vi "PID control - Copy.vi"() -> ()   [LabVIEW 2017]
uses:
  <vilib>/Simulation/Scripting/Companion Diagram/SimConfigNode/SimParams.ctl
  <vilib>/Simulation/Scripting/Companion Diagram/SimConfigNode/_simSolvers.ctl
  <vilib>/Simulation/Implementation/Shared/SIMSCR Execution Mode.ctl
  <vilib>/Simulation/Param Hierarchy/Typedefs/SIMPH Param Control Actions.ctl
  <vilib>/Simulation/Implementation/Shared/NILVSim_ParamChanged.vi
  <vilib>/Simulation/Implementation/Shared/NILVSIM_BeginStep.vi
  <vilib>/Simulation/Implementation/Shared/NILVSim_Manager.vi
  <vilib>/Utility/error.llb/Clear Errors.vi
  <vilib>/Simulation/Implementation/Shared/NILVSim_FinalizeModel.vi
  <vilib>/DAQmx/read.llb/DAQmx Read (Counter DBL 1Chan 1Samp).vi
  <vilib>/DAQmx/read.llb/DAQmx Read (Digital Bool 1Line 1Point).vi
  917b7e52-755f-4d44-bea8-9e7c9beac24e.vi
  a58f9967-76f1-4ebc-ad3d-26e75a3ca160.vi
  <vilib>/DAQmx/write.llb/DAQmx Write (Analog DBL 1Chan 1Samp).vi
  <vilib>/DAQmx/create/channels.llb/DAQmx Create Channel (AO-Voltage-Basic).vi
  <vilib>/DAQmx/create/channels.llb/DAQmx Create Channel (DI-Digital Input).vi
  <vilib>/DAQmx/create/channels.llb/DAQmx Create Channel (CI-Count Edges).vi
  <vilib>/Simulation/Implementation/Shared/SIM Unbundle Sim Info.vi
  <vilib>/Simulation/Implementation/Shared/NILVSim_Initialize.vi
  <vilib>/Simulation/Utility/Implementation/NILVSim Get Time and IsAcceptedStep.vi
  <vilib>/Simulation/Implementation/Shared/SIMSH Read Queue.vi
  <vilib>/Simulation/Implementation/Shared/NILVSim_GetModelError.vi
  <vilib>/Simulation/Implementation/Shared/SIM Bundle Sim Info.vi
  <vilib>/DAQmx/miscellaneous.llb/DAQmx Fill In Error Info.vi
  <vilib>/Simulation/Implementation/XNodeFramework/SimXNode/SimX.xnode
  <vilib>/Simulation/Model Libraries/PID/SIM PID (Parallel).vi
  <vilib>/Simulation/Model Libraries/PID/SIM PID.vi
  <vilib>/Simulation/Scripting/Companion Diagram/SimConfigNode/SimDog.xnode
  <vilib>/Simulation/Model Libraries/PID/SIM PID (Academic).vi
  <vilib>/Simulation/Implementation/Shared/NI_SIM_Implementation.lvlib
panel:
  out "resetting x":bool
  out "resetting y":bool
  out "index":dbl
  out "x check":dbl
  out "stop":bool
  out "y final check":dbl
  out "y check":dbl
  out "array x Length":dbl
  out "X array":dbl[](array[numeric])
  out "array Y length":dbl
  out "Y array":dbl[](array[numeric])
  out "Numeric y":dbl
  out "Numeric x":dbl
  out "Numeric 2":dbl
  in  "Radius":dbl
  out "led check":bool
  in  "check instruc":bool
  out "down 2":bool
  out "down":bool
  out "right":bool
  out "x entered":dbl
  out "y enetred":dbl
  out "greater -1 x":bool
  out "less 1 x":bool
  out "direction selected":dbl
  out "circle reset":bool
  in  "part circle":T1(ring)=enum."a"
  out "at 2f":bool
  out "Step 2J":bool
  out "Step 2H":bool
  out "Shape drawing steps":enum16{"corner", "1st switch", "reverse"}(ring)
  out "Step 2D":bool
  out "Step 2C":bool
  out "c":bool
  in  "height":dbl
  in  "length":dbl
  in  "part":T2(ring)=enum."a"
  out "Step 2A":bool
  out "Step 2B":bool
  in  "Has encoders been reset?":enum16{"don't reset", "reset"}(ring)
  out "x distance currently being travelled":dbl
  out "y distance currently being travelled":dbl
  out "error calced":dbl
  out "p1 dis 2":dbl
  out "p1 dis":dbl
  out "error y":dbl
  out "calc distance y":dbl
  out "calc distanc x":dbl
  out "error x":dbl
  out "reached y":bool
  out "reached x":bool
  out "Numeric":dbl
  in  "Draw rectangle":bool
  in  "Draw circle":bool
  out "In drawing mode":bool
  in  "Right-Down":bool
  in  "Left-Up":bool
  in  "Left-Down":bool
  in  "Right-Up":bool
  in  "right":bool
  in  "left":bool
  in  "motor 2":dbl(slide)=1.5 scale=-10.0..10.0
  in  "down":bool
  in  "up":bool
  in  "Y Length":dbl=30.0
  in  "X Length":dbl=30.0
  in  "Motor 2 encoder":tag="Dev1/ctr1"
  out "Pulses M2":dbl format="%.2f"
  in  "Motor 1 encoder":tag="Dev1/ctr0"
  out "Pulses M1":dbl format="%.2f"
  out "Right":bool
  out "Bottom":bool
  out "Left":bool
  out "Top":bool
  in  "Switch 4/Line 3":tag="Dev1/port0/line3"
  in  "Switch 3/Line 2":tag="Dev1/port0/line2"
  in  "Switch 2/Line 1":tag="Dev1/port0/line1"
  in  "Switch 1/Line 0":tag="Dev1/port0/line0"
  in  "Motor stop":bool
  in  "Motor 1":tag="Dev1/ao0"
  in  "max Voltage":dbl=10.0
  in  "Min Voltage":dbl=-10.0
  in  "Motor 2":tag="Dev1/ao1"
  in  "motor 1":dbl(slide)=1.5 scale=-10.0..10.0
  in  "stop":bool
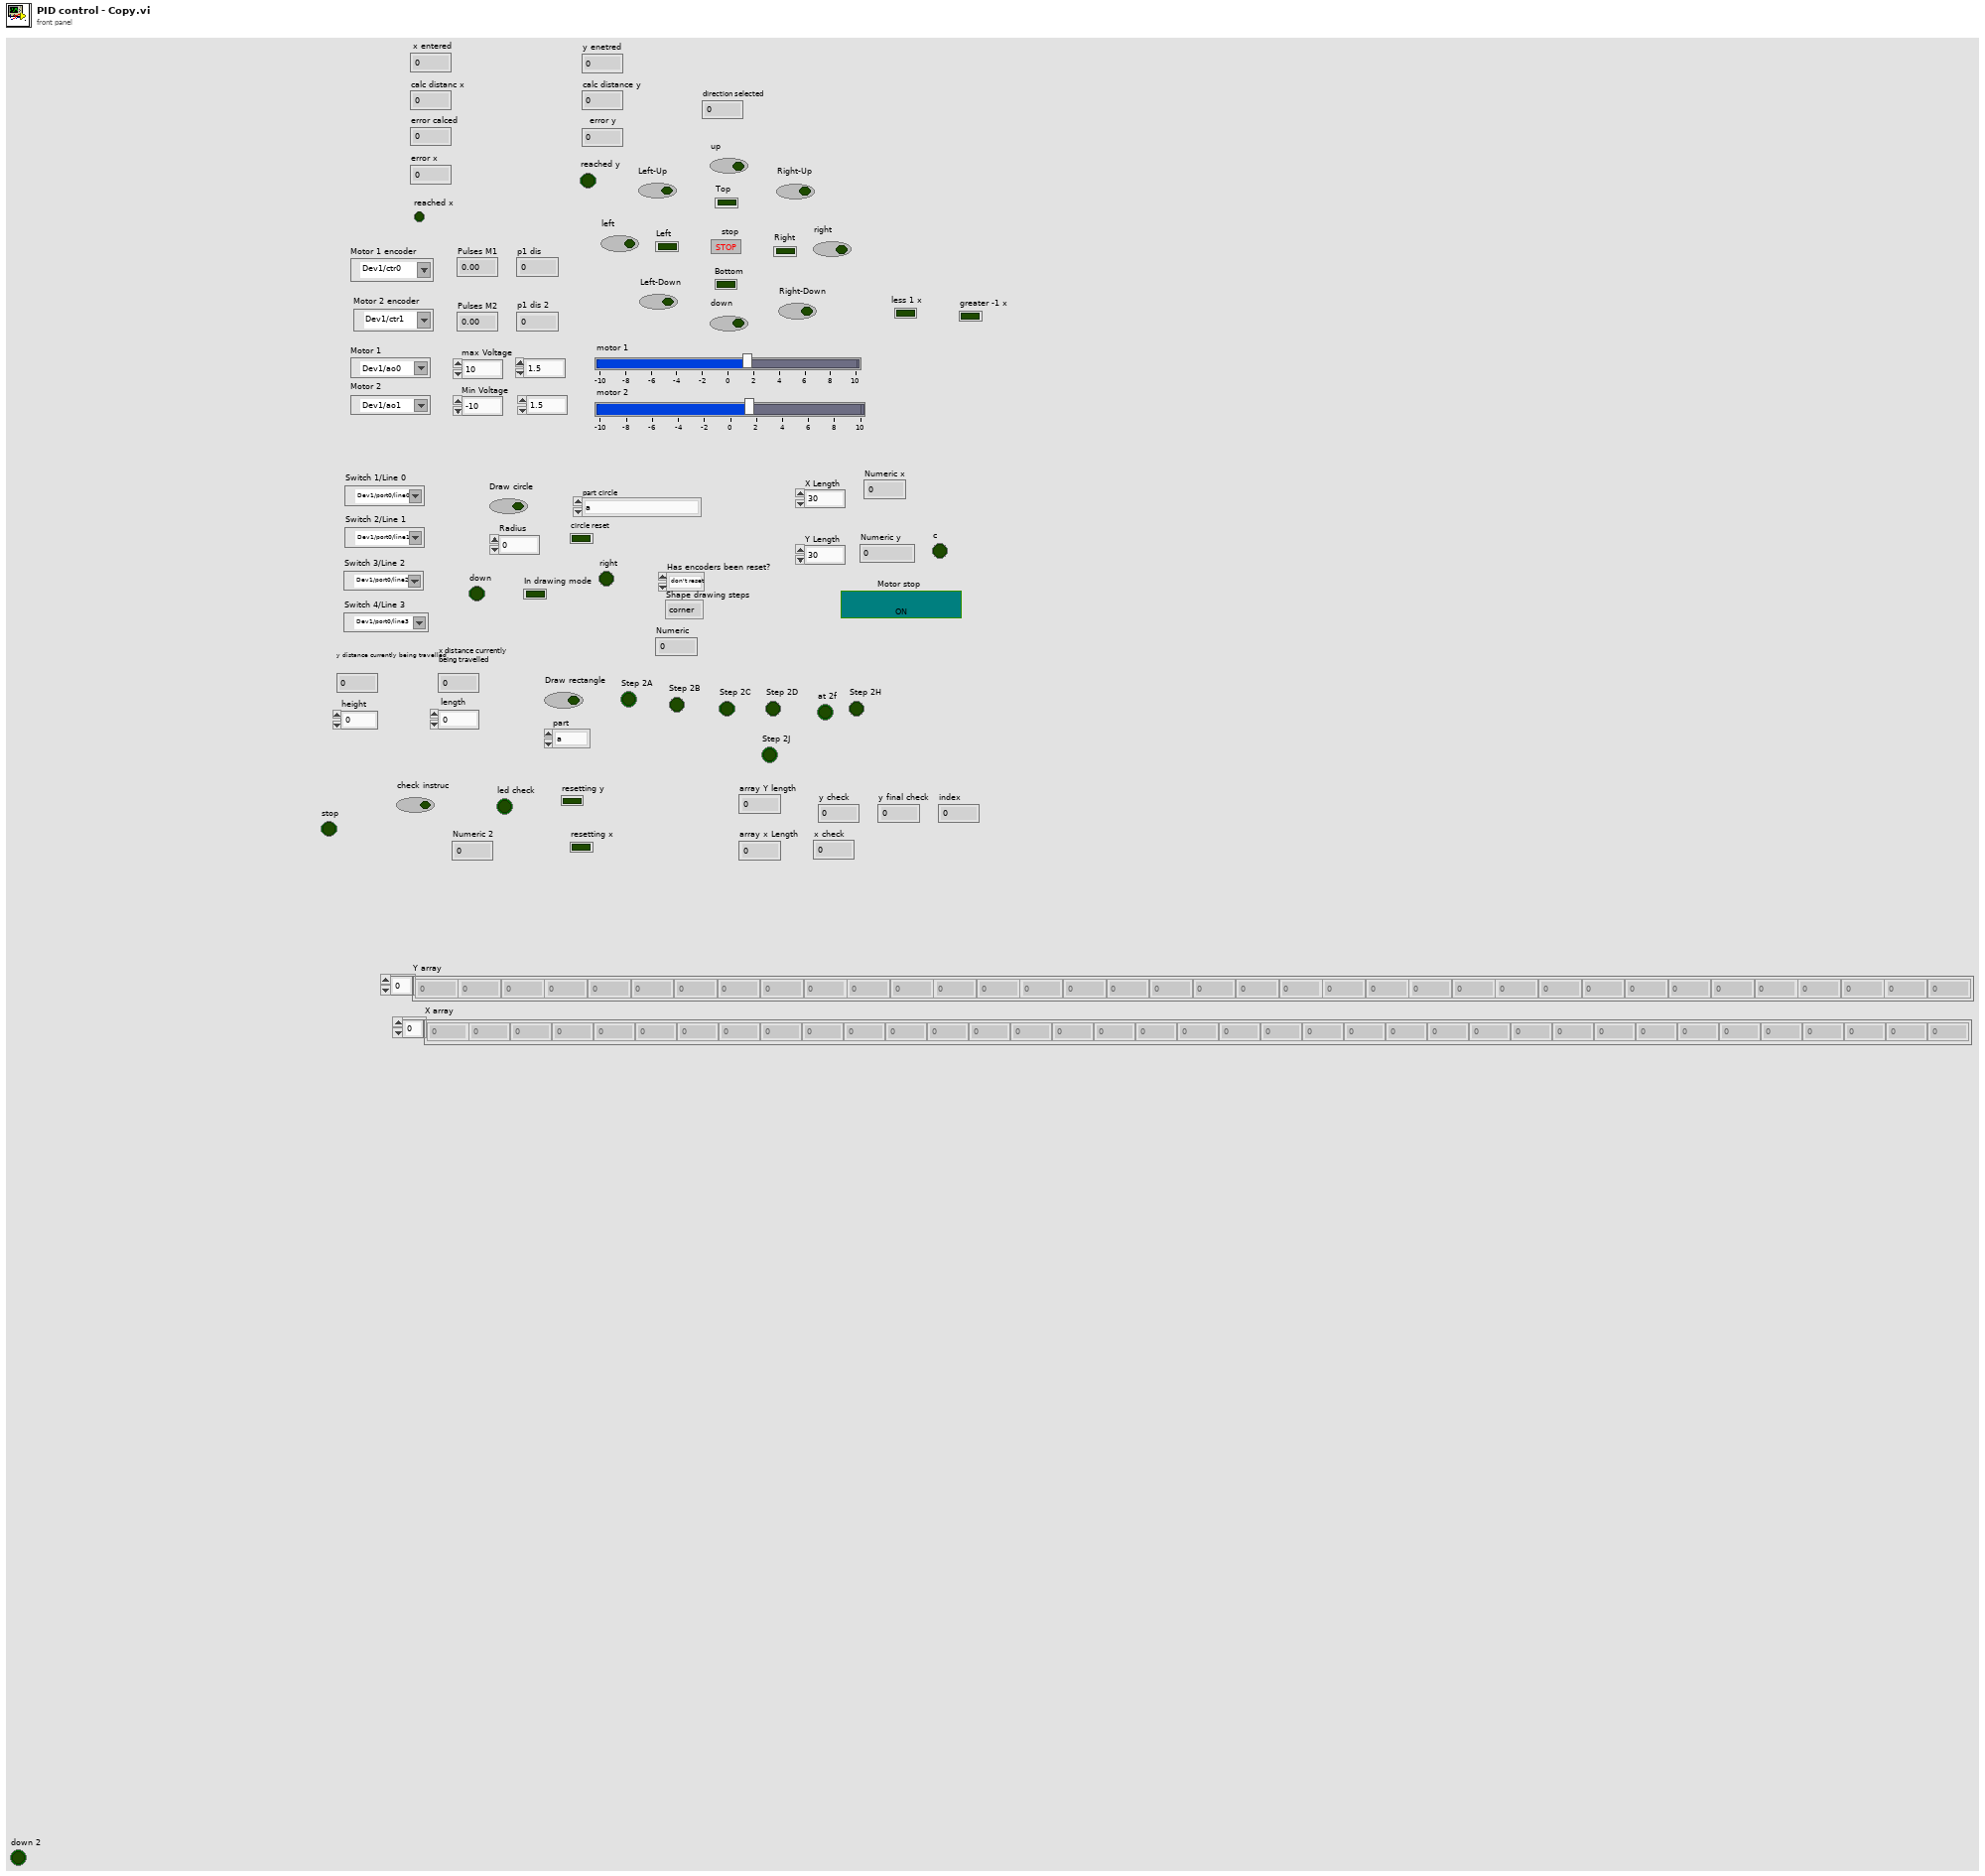
[diagram p1: front panel]
types:
  T1 = enum16{"nothing", "circle", "reset_before_circle", "radius_travel", "going right", "going down", "a"}
  T2 = enum16{"nothing", "j", "i", "h", "g", "f", "e", "d", "c", "b", "a"}
  T3 = enum16{"Simulate to Completion", "Single Time-Step Simulation (Fixed Step Only)"}
  T4 = typedef "SIMSCR Execution Mode.ctl" = enum16{"Simulate to Completion", "Single Time-Step Simulation (Fixed Step Only)"}
  T5 = typedef "SIMPH Param Control Actions.ctl" = enum16{"get params", "set params"}
  T6 = cluster{"SIMSH Sim Time":dbl, "SIM PID Derivative Gain.vi":cluster{"output":dbl}, "SIM PID Derivative Gain.vi - SIMSH":cluster{"SIMSH Sim Time":dbl, "t 3":dbl, "Select 2":cluster{"s? t:f":dbl}, "Equal?":cluster{"x = y?":bool}, "Or":cluster{"x .or. y?":bool}, "Equal To 0?":cluster{"x = 0?":bool}}, "High Frequency [s] (Tf)":dbl, "Gain":cluster{"output":dbl}, "Summation":cluster{"Result":dbl}, "Integral Gain - series.vi":cluster{"output":dbl}, "Integral Gain - series.vi - SIMSH":cluster{"SIMSH Sim Time":dbl, "Select 2":cluster{"s? t:f":dbl}, "integral in gain?":bool, "Integrator":cluster{"output y(t)":dbl}, "Gain 2":cluster{"output":dbl}, "Select":cluster{"s? t:f":dbl}, "Equal To 0?":cluster{"x = 0?":bool}, "Reciprocal":cluster{"1/x":dbl}}}
  T7 = typedef "SimParams.ctl" = cluster{"Initial Time (s)":dbl, "Final Time (s)":dbl, "Step Size (s)":dbl, "ODE Solver":T8, "Minimum Step Size (s)":dbl, "Maximum Step Size (s)":dbl, "Relative Tolerance":dbl, "Absolute Tolerance":dbl, "Software Timing":bool, "Initial Step Size (s)":dbl, "Automatic Fixed Step Size?":bool, "Automatic Discrete Step Size?":bool, "Discrete Step Size (s)":dbl, "Calculate using Time Step":bool, "Solver Wired?":bool, "Prev.Frm.Expected End":u64, "Prev.Frm.Actual End":u64, "Prev.Frm.Finished Late?":bool, "Prev.Iter.Expected End":u64, "Prev.Iter.Actual End":u64, "Prev.Iter.Finished Late?":bool, "Expected Iteration Start":u64, "Actual Iteration Start":u64, "Expected Frame Start":u64, "Actual Frame Start":u64, "Source Name":string, "Name":string, "Period":i64, "Deadline":i64, "Offset":i64, "Start":i64, "Priority":i32, "Timeout":i32, "Processor":i32, "Mode":enum32{"No Change", "Process missed periods, maintain original phase", "Discard missed periods, maintain original phase", "Process missed periods, ignore original phase", "Discard missed periods, ignore original phase"}, "Wakeup reason":enum32{"Normal", "Aborted", "Asynchronous wakeup", "Timing source error", "Timed loop error", "Timeout"}, "Error":errorcluster, "Source Type":string, "Secondary Source Type":string, "Global End Time":u64, "Global Start Time":u64, "Full Solver Reset":bool, "Execution Mode":T4, "Nan/Inf Check":bool, "Custom Solver Library":string, "Solver Is Variable":bool, "custom solver name":string, "Signal Collection Decimation":u32}
  T8 = typedef "_simSolvers.ctl" = enum16{"Runge-Kutta 1 (Euler)", "Runge-Kutta 2", "Runge-Kutta 3", "Runge-Kutta 4", "Runge-Kutta 23 (variable)", "Runge-Kutta 45 (variable)", "BDF (variable)", "Adams-Moulton (variable)", "Rosenbrock (variable)", "Discrete States Only", "SDIRK 4 (variable)", "Radau 5 (variable)", "Radau 9 (variable)", "Radau 13 (variable)", "Radau [Variable Order] (variable)", "Gear's Method (variable)", "Linearizer", "State Query", "Trim Eval", "Custom Solver"}
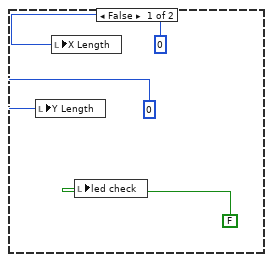
[diagram p2: hidden frame]
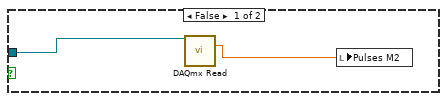
[diagram p3: hidden frame]
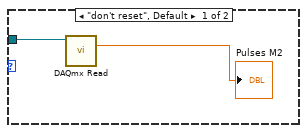
[diagram p4: hidden frame]
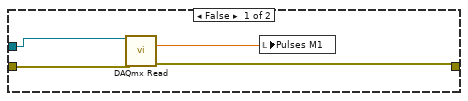
[diagram p5: hidden frame]
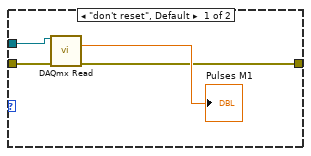
[diagram p6: hidden frame]
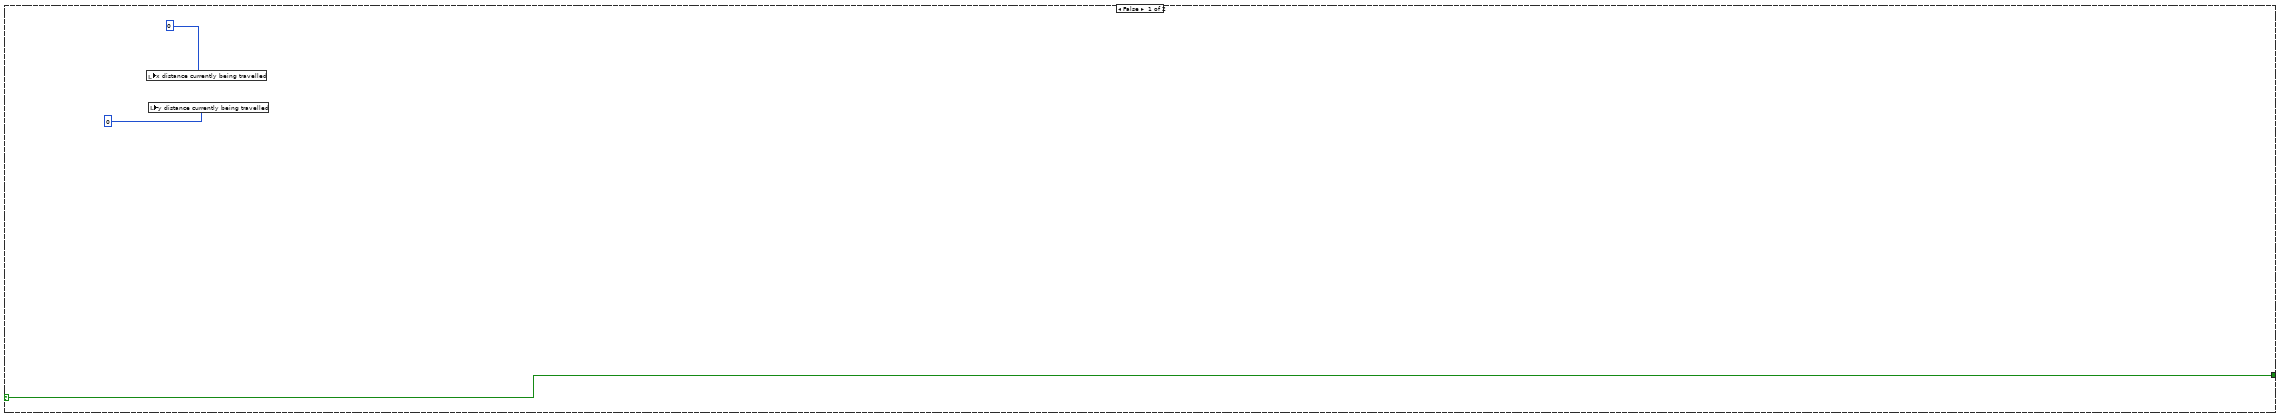
[diagram p7: hidden frame]
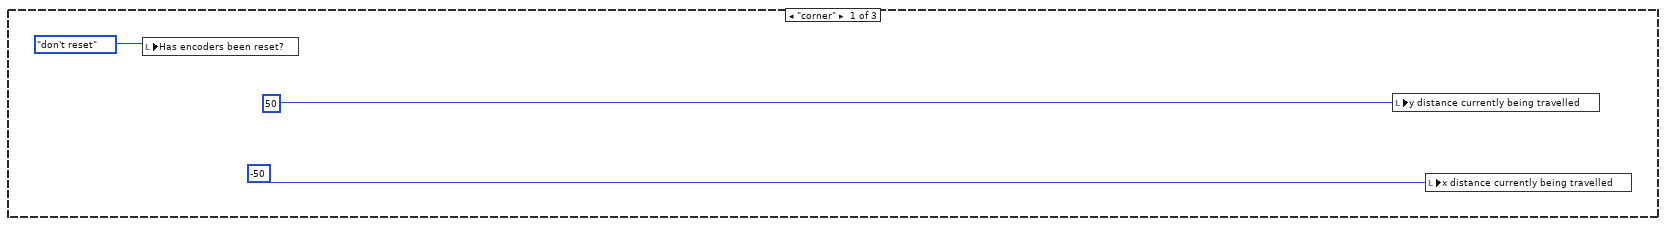
[diagram p8: hidden frame]
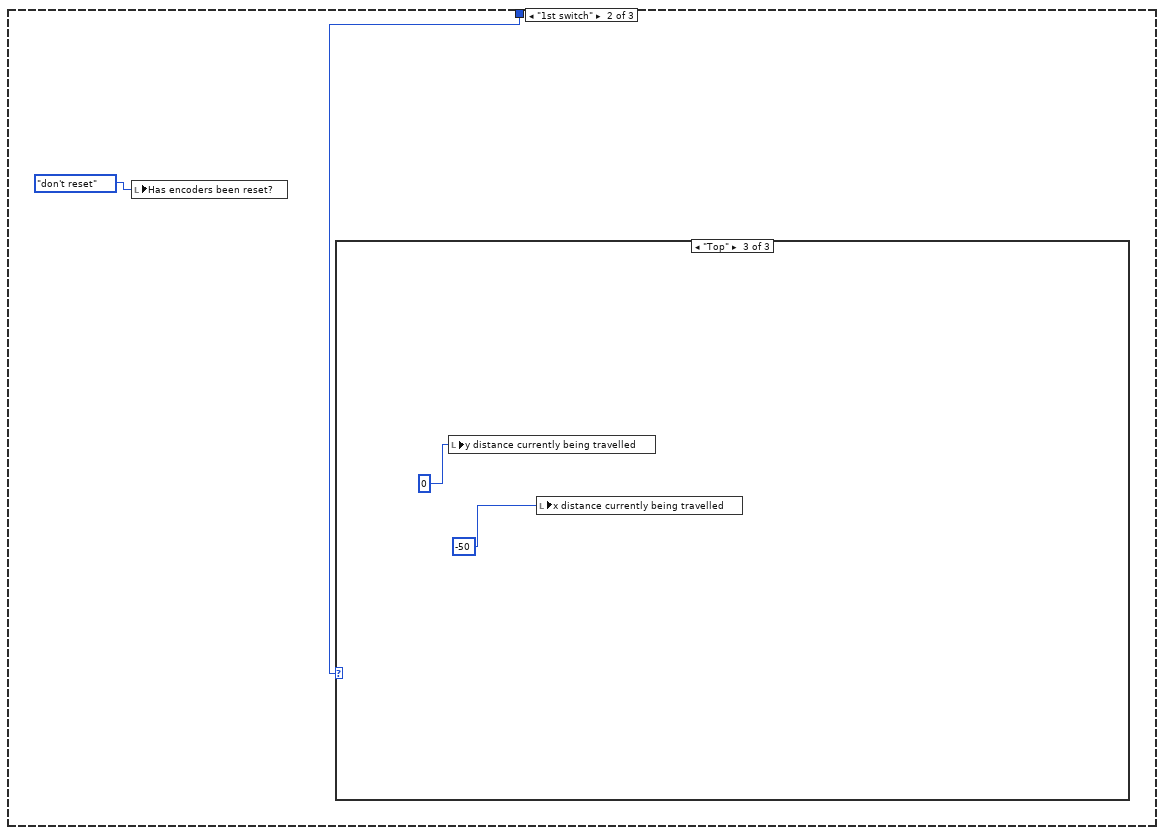
[diagram p9: hidden frame]
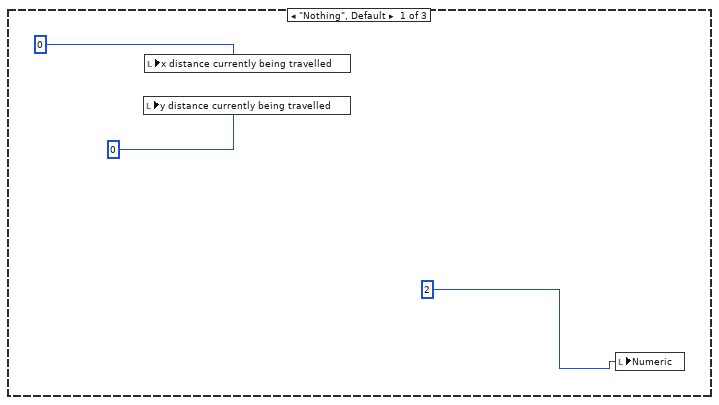
[diagram p10: hidden frame]
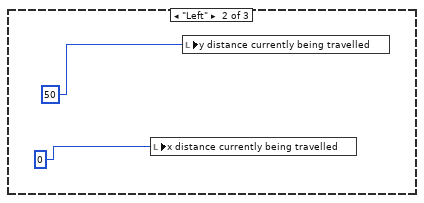
[diagram p11: hidden frame]
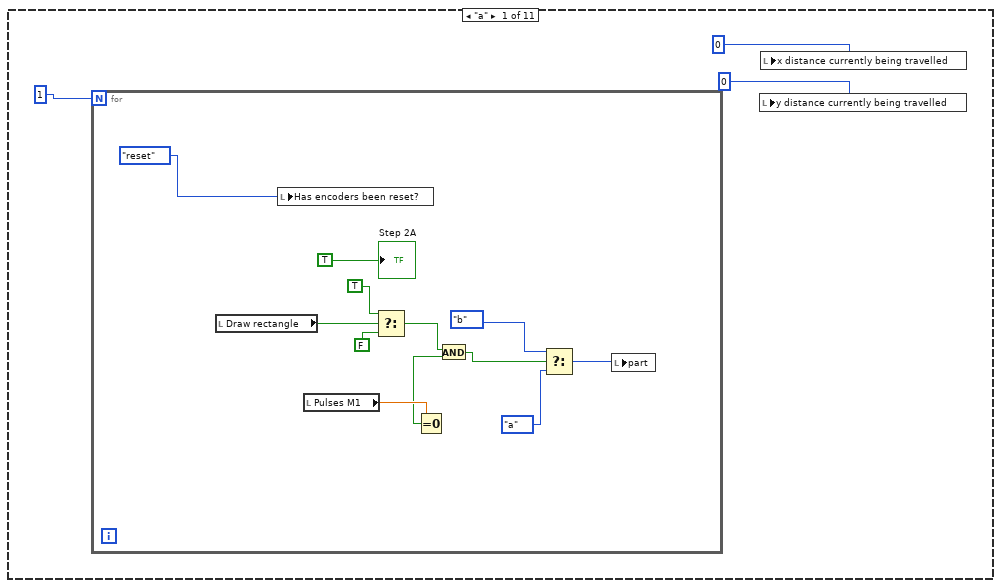
[diagram p12: hidden frame]
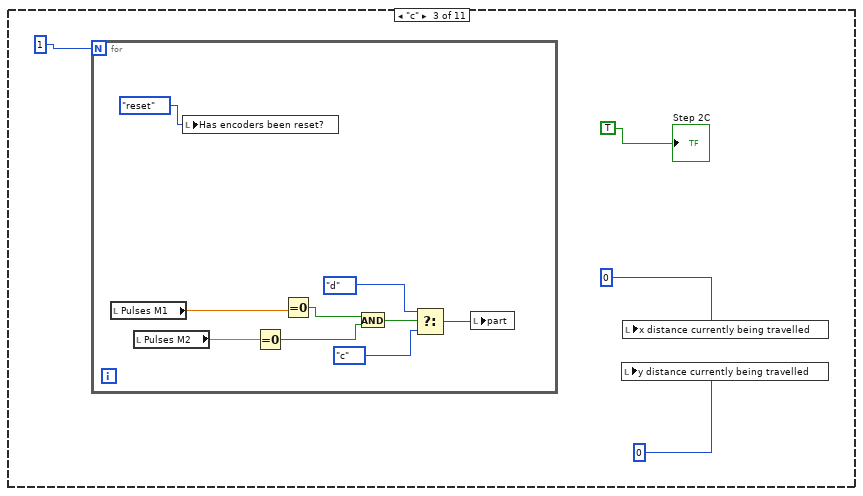
[diagram p13: hidden frame]
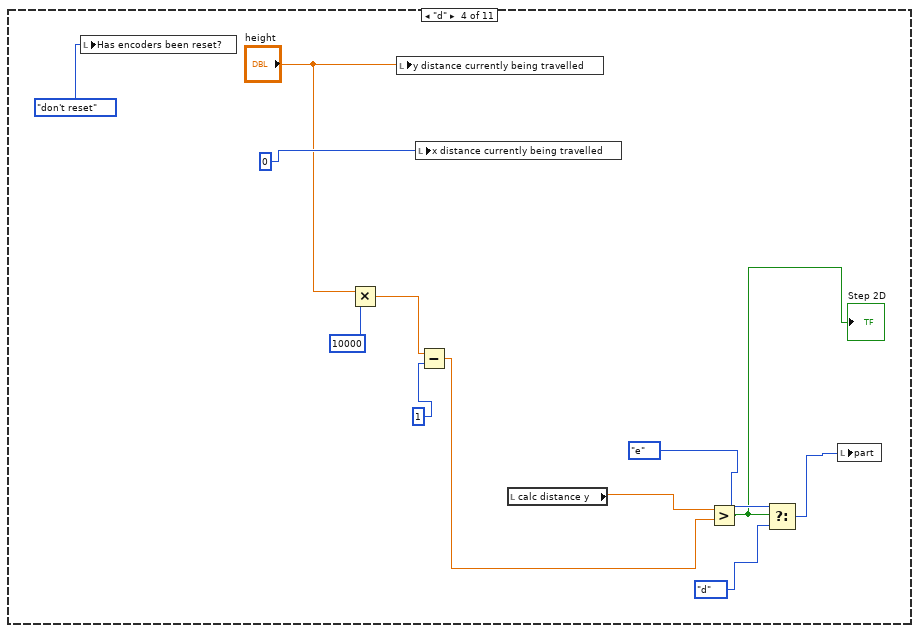
[diagram p14: hidden frame]
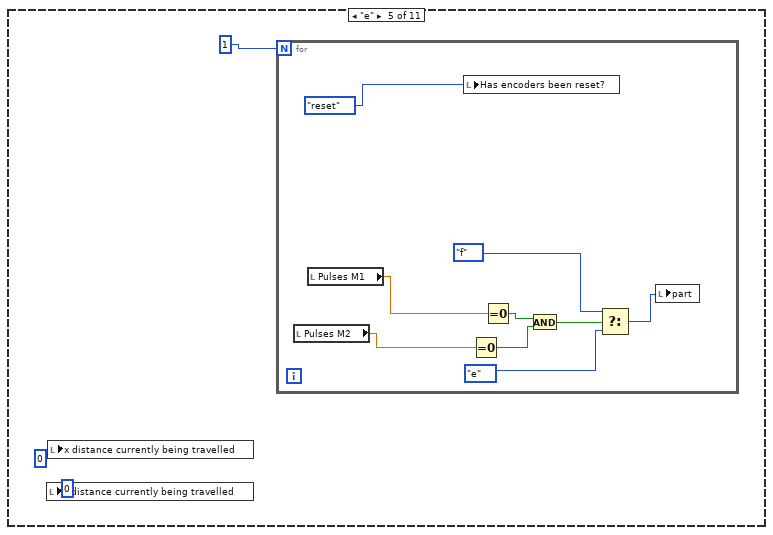
[diagram p15: hidden frame]
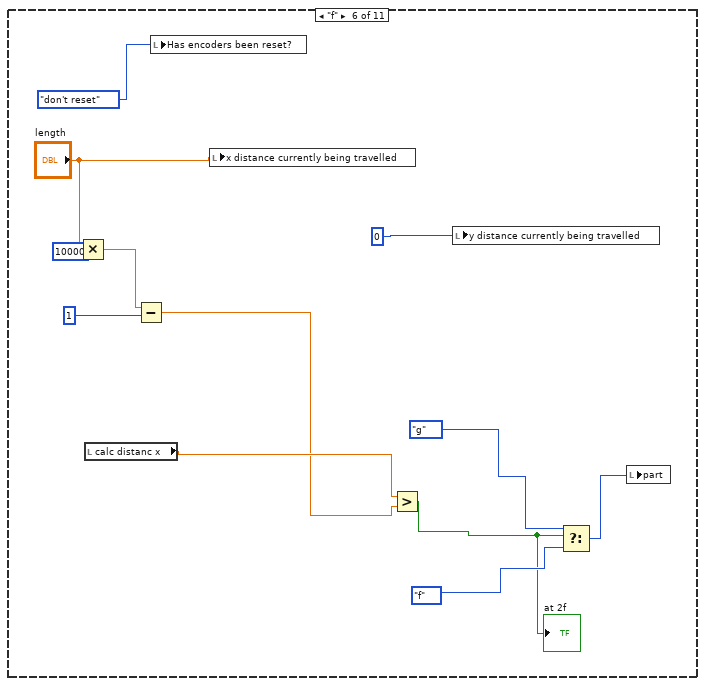
[diagram p16: hidden frame]
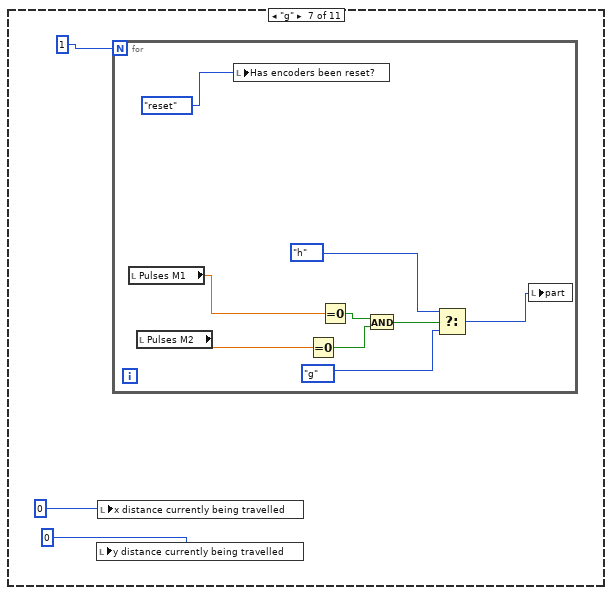
[diagram p17: hidden frame]
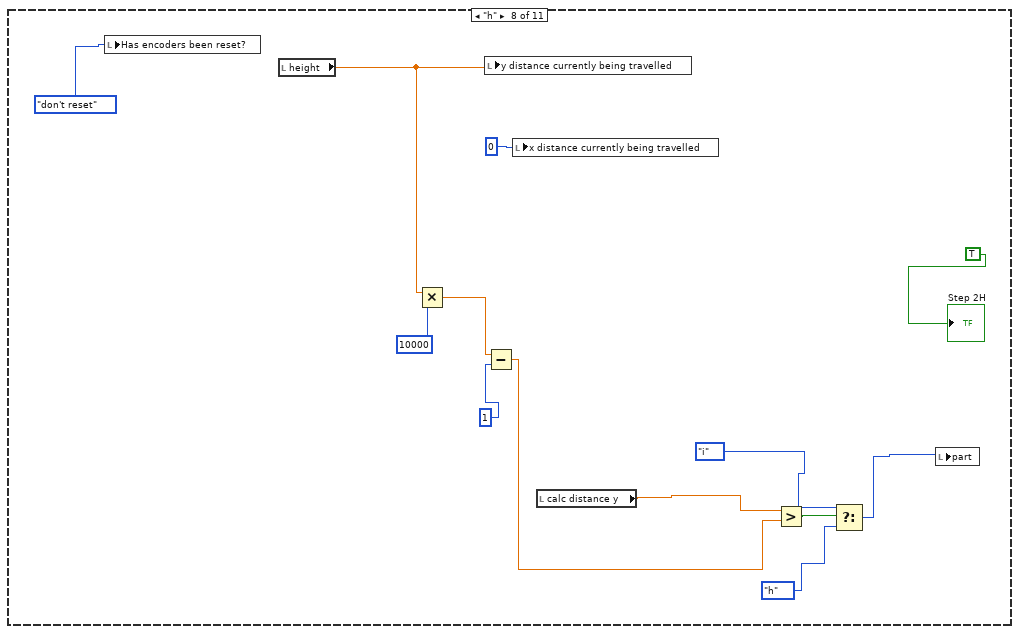
[diagram p18: hidden frame]
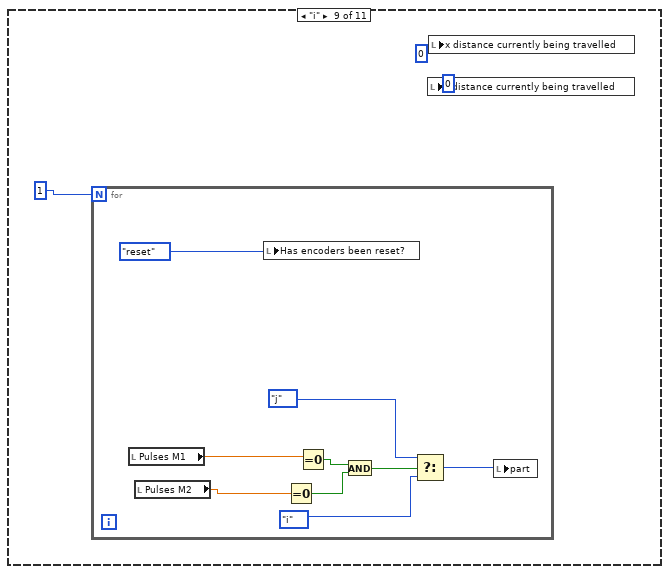
[diagram p19: hidden frame]
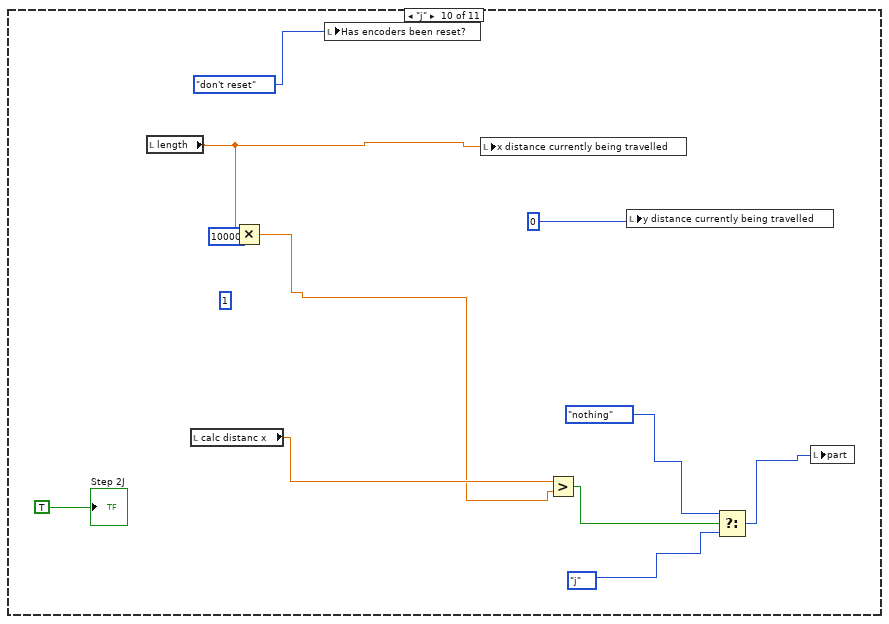
[diagram p20: hidden frame]
diagram:
  n1 = call-poly <vilib>:"DAQmx Create Virtual Channel.vi"("lines"="Switch 1/Line 0") -> ("task out"=w36:refnum<k21>, "error out"=w32:errorcluster)  [unwired: 13 in]
  n2 = call-poly <vilib>:"DAQmx Create Virtual Channel.vi"("lines"="Switch 2/Line 1") -> ("task out"=w35:refnum<k21>, "error out"=w31:errorcluster)  [unwired: 13 in]
  n3 = call-poly <vilib>:"DAQmx Create Virtual Channel.vi"("lines"="Switch 3/Line 2") -> ("task out"=w34:refnum<k21>, "error out"=w30:errorcluster)  [unwired: 13 in]
  n4 = call-poly <vilib>:"DAQmx Create Virtual Channel.vi"("lines"="Switch 4/Line 3") -> ("task out"=w33:refnum<k21>, "error out"=w29:errorcluster)  [unwired: 13 in]
  n5 = call <vilib>:"DAQmx Start Task.vi"("task/channels in"=w36, "error in"=w32) -> ("task out"=w28:refnum<k21>, "error out"=w26:errorcluster)  [unwired: 12 in]
  n6 = call <vilib>:"DAQmx Start Task.vi"("task/channels in"=w35, "error in"=w31) -> ("task out"=w24:refnum<k21>, "error out"=w21:errorcluster)  [unwired: 12 in]
  n7 = call <vilib>:"DAQmx Start Task.vi"("task/channels in"=w34, "error in"=w30) -> ("task out"=w23:refnum<k21>, "error out"=w20:errorcluster)  [unwired: 12 in]
  n8 = call <vilib>:"DAQmx Start Task.vi"("task/channels in"=w33, "error in"=w29) -> ("task out"=w22:refnum<k21>, "error out"=w19:errorcluster)  [unwired: 12 in]
  n9 = call-poly <vilib>:"DAQmx Create Virtual Channel.vi"("maximum value"="max Voltage", "minimum value"="Min Voltage", "physical channels"="Motor 1") -> ("task out"=w46:refnum<k21>, "error out"=w42:errorcluster)  [unwired: 11 in]
  n10 = call-poly <vilib>:"DAQmx Create Virtual Channel.vi"("counter"="Motor 2 encoder") -> ("task out"=w6:refnum<k21>)  [unwired: 13 in, 1 out]
  n11 = call-poly <vilib>:"DAQmx Create Virtual Channel.vi"("maximum value"="max Voltage", "minimum value"="Min Voltage", "physical channels"="Motor 2") -> ("task out"=w49:refnum<k21>, "error out"=w41:errorcluster)  [unwired: 11 in]
  n12 = call-poly <vilib>:"DAQmx Create Virtual Channel.vi"("counter"="Motor 1 encoder") -> ("task out"=w7:refnum<k21>, "error out"=w2:errorcluster)  [unwired: 13 in]
  n13 = call <vilib>:"DAQmx Start Task.vi"("task/channels in"=w6) -> ("task out"=w1:refnum<k21>)  [unwired: 13 in, 1 out]
  n14 = call <vilib>:"DAQmx Start Task.vi"("task/channels in"=w7) -> ("task out"=w3:refnum<k21>)  [unwired: 13 in, 1 out]
  n15 = while {
    tunnel: w49 -> [w236]
    tunnel: [w233] -> w48
    tunnel: w46 -> [w230]
    tunnel: [w229] -> w45
    tunnel: w42 -> [w227]
    tunnel: w41 -> [w226]
    tunnel: w28 -> [w220]
    tunnel: [w219] -> w27
    tunnel: w26 -> [w218]
    tunnel: [w217] -> w25
    tunnel: w24 -> [w216]
    tunnel: w23 -> [w215]
    tunnel: w22 -> [w214]
    tunnel: w21 -> [w213]
    tunnel: w20 -> [w212]
    tunnel: w19 -> [w211]
    tunnel: [w210] -> w18
    tunnel: [w209] -> w17
    tunnel: [w208] -> w16
    tunnel: [w207] -> w15
    tunnel: [w206] -> w14
    tunnel: [w205] -> w13
    tunnel: [w139] -> w10
    tunnel: w3 -> [w141]
    tunnel: w2 -> [w140]
    tunnel: w1 -> [w137]
    stop <- "stop" stop-if-true
    (unwired) TRUE
    n16 = Or(x="Draw circle", y="Draw rectangle") -> (x .or. y?=w149:bool)
    n17 = case shown="True" "check instruc" {
      frame False {
        n18 = local write "Y Length"(0) -> ()
        n19 = local write "X Length"(0) -> ()
        n20 = local write "led check"(FALSE) -> ()
      }
      frame True {
        n21 = flat-sequence {
          frame #0 {
            n22 = while {
              stop <- w247 stop-if-true
              n23 = for {
                N: 50 -> [_]
                shift-right: [w253] -> w246
                shift-left: _ -> [_]
                tunnel: [w253] -> w241 mode=indexing
                shift-right: [w252] -> w244
                shift-left: _ -> [_]
                tunnel: [w252] -> w242 mode=indexing
                i -> [w255]
                n24 = Multiply(x=2, y=3.141592653589793) -> (x*y=w259:dbl)
                n25 = Increment(x=w255) -> (x+1=w257:i32)
                n26 = Divide(x=w259, y=50) -> (x/y=w261:dbl)
                n27 = Multiply(x=w261, y=w257) -> (x*y=w258:dbl)
                n28 = local write "led check"(TRUE) -> ()
                n29 = local write "Has encoders been reset?"(enum16{"don't reset", "reset"}."don't reset") -> ()
                n30 = Cosine(x=w258) -> (cos(x)=w264:dbl)
                n31 = Sine(x=w258) -> (sin(x)=w265:dbl)
                n32 = Multiply(x=w265, y="Radius") -> (x*y=w253:dbl)
                n33 = Multiply(x=w264, y="Radius") -> (x*y=w252:dbl)
                "Numeric 2" <- w255
              }
              "Numeric y" <- w246
              "Y array" <- w241
              "Numeric x" <- w244
              "X array" <- w242
              n34 = local read "Numeric 2"() -> (w249:dbl)
              n35 = Equal?(x=w249, y=49) -> (x = y?=w247:bool)
              n36 = Array Size(array=w241) -> (size(s)=→"array Y length":i32)
              n37 = Array Size(array=w242) -> (size(s)=→"array x Length":i32)
            }
            n38 = local write "index"(0) -> ()
          }
          frame #1 {
            n39 = flat-sequence {
              tunnel: [w272] -> w271
              tunnel: w268 -> [w272]
              tunnel: w271 -> [w284]
              tunnel: [w286] -> w270
              tunnel: [w285] -> w266
              tunnel: [w296] -> w269
              tunnel: w266 -> [w296]
              frame #0 {
                n40 = local read "Y array"() -> (w276:dbl[])
                n41 = local read "X array"() -> (w274:dbl[])
                n42 = Index Array(array=w274, index=w272) -> (element=→"x check":dbl)
                n43 = Index Array(array=w276, index=w272) -> (element=→"y check":dbl)
              }
              frame #1 {
                n44 = local read "calc distance y"() -> (w293:dbl)
                n45 = local read "calc distanc x"() -> (w289:dbl)
                n46 = local read "resetting y"() -> (w278:bool)
                n47 = local read "resetting x"() -> (w277:bool)
                n48 = Greater?(x=w293, y=1000) -> (0:→"resetting y":bool)
                n49 = Greater?(x=w289, y=1000) -> (0:→"resetting x":bool)
                n50 = local read "index"() -> (w283:dbl)
                n51 = And(x=w278, y=w277) -> (x .and. y?=w287:bool)
                n52 = Add(x=1, y=w283) -> (x+y=w281:dbl)
                n53 = Select(t=w281, s=w287, f=w284) -> (s? t:f=w285:dbl)
                "y final check" <- w285
                n54 = Equal?(x=w285, y=50) -> (x = y?=w286:bool)
                "led check" <- TRUE
              }
              frame #2 {
                n55 = local write "resetting x"(FALSE) -> ()
                n56 = local write "resetting y"(FALSE) -> ()
              }
            }
            n57 = feedback-in #1(w269) -> ()
            n58 = feedback #1() -> (w268:dbl)  [unwired: 1 in]
            "index" <- w268
            n59 = local write "Has encoders been reset?"(enum16{"don't reset", "reset"}."don't reset") -> ()
            "stop" <- w270
          }
        }
      }
    }
    n60 = local read "error y"() -> (w108:dbl)
    n61 = local read "error y"() -> (w107:dbl)
    n62 = local read "error x"() -> (w109:dbl)
    n63 = local read "error y"() -> (w123:dbl)
    n64 = local read "error y"() -> (w120:dbl)
    n65 = local read "error x"() -> (w116:dbl)
    n66 = local read "error x"() -> (w115:dbl)
    n67 = local read "error y"() -> (w124:dbl)
    n68 = local read "error x"() -> (w125:dbl)
    n69 = Less Than 0?(x=w108) -> (x < 0?=w106:bool)
    n70 = Less Than 0?(x=w109) -> (x < 0?=w105:bool)
    n71 = Greater Than 0?(x=w107) -> (x > 0?=w104:bool)
    n72 = Less Than 0?(x=w120) -> (x < 0?=w118:bool)
    n73 = Equal To 0?(x=w125) -> (x = 0?=w119:bool)
    n74 = Greater Than 0?(x=w123) -> (x > 0?=w122:bool)
    n75 = local read "error y"() -> (w101:dbl)
    n76 = local read "error x"() -> (w100:dbl)
    n77 = Greater Than 0?(x=w116) -> (x > 0?=w114:bool)
    n78 = Equal To 0?(x=w124) -> (x = 0?=w113:bool)
    n79 = Less Than 0?(x=w115) -> (x < 0?=w112:bool)
    n80 = And(x=w106, y=w105) -> (x .and. y?=w102:bool)
    n81 = And(x=w105, y=w104) -> (x .and. y?=w103:bool)
    n82 = And(x=w122, y=w119) -> (x .and. y?=w121:bool)
    n83 = And(x=w119, y=w118) -> (x .and. y?=w117:bool)
    n84 = local read "error y"() -> (w96:dbl)
    n85 = And(x=w114, y=w113) -> (x .and. y?=w111:bool)
    n86 = And(x=w113, y=w112) -> (x .and. y?=w110:bool)
    n87 = Greater Than 0?(x=w101) -> (x > 0?=w99:bool)
    n88 = Greater Than 0?(x=w100) -> (x > 0?=w97:bool)
    n89 = Less Than 0?(x=w96) -> (x < 0?=w95:bool)
    n90 = And(x=w99, y=w97) -> (x .and. y?=w98:bool)
    n91 = And(x=w97, y=w95) -> (x .and. y?=w94:bool)
    n92 = Select(t=1, s=w121, f=0) -> (s? t:f=w189:i32)
    n93 = Select(t=10, s=w110, f=0) -> (s? t:f=w187:i32)
    n94 = Select(t=2, s=w117, f=0) -> (s? t:f=w188:i32)
    n95 = Select(t=100, s=w98, f=0) -> (s? t:f=w185:i32)
    n96 = Select(t=200, s=w102, f=0) -> (s? t:f=w184:i32)
    n97 = Select(t=20, s=w111, f=0) -> (s? t:f=w186:i32)
    n98 = Select(t=1000, s=w103, f=0) -> (s? t:f=w183:i32)
    n99 = Select(t=2000, s=w94, f=0) -> (s? t:f=w169:i32)
    n100 = Add(x=w189, y=w188) -> (x+y=w182:i32)
    n101 = Add(x=w187, y=w186) -> (x+y=w181:i32)
    n102 = Add(x=w185, y=w184) -> (x+y=w180:i32)
    n103 = Add(x=w183, y=w169) -> (x+y=w168:i32)
    n104 = local read "y check"() -> (w51:dbl)
    n105 = Add(x=w182, y=w181) -> (x+y=w179:i32)
    n106 = Add(x=w180, y=w168) -> (x+y=w167:i32)
    n107 = call-poly <vilib>:"DAQmx Read.vi"("task/channels in"=w220, "error in"=w218) -> ("task out"=w219:refnum<k21>, "data"=w151:bool, "error out"=w217:errorcluster)  [unwired: 11 in]
    "Top" <- w151
    n108 = call-poly <vilib>:"DAQmx Read.vi"("task/channels in"=w216, "error in"=w213) -> ("task out"=w210:refnum<k21>, "data"=w160:bool, "error out"=w207:errorcluster)  [unwired: 11 in]
    "Bottom" <- w160
    n109 = call-poly <vilib>:"DAQmx Read.vi"("task/channels in"=w215, "error in"=w212) -> ("task out"=w209:refnum<k21>, "data"=w159:bool, "error out"=w206:errorcluster)  [unwired: 11 in]
    "Right" <- w159
    n110 = call-poly <vilib>:"DAQmx Read.vi"("task/channels in"=w214, "error in"=w211) -> ("task out"=w208:refnum<k21>, "data"=w158:bool, "error out"=w205:errorcluster)  [unwired: 11 in]
    "Left" <- w158
    n111 = Add(x=w179, y=w167) -> (x+y=w93:i32)
    "direction selected" <- w93
    n112 = local read "check instruc"() -> (w52:bool)
    n113 = Select(t=w51, s=w52, f="Y Length") -> (s? t:f=w53:dbl)
    n114 = Multiply(x=w53, y=10) -> (x*y=w55:dbl)
    "y enetred" <- w55
    n115 = local read "Pulses M1"() -> (w138:dbl)
    n116 = local read "Pulses M2"() -> (w142:dbl)
    n117 = Divide(x=w138, y=52.56) -> (x/y=→"p1 dis":dbl)
    n118 = feedback #2() -> (w67:dbl)  [unwired: 1 in]
    "calc distance y" <- w67
    n119 = formula code="if (Ylength==0)\nYerror=0;\n else  \nif(Ylength<0)\nYerror= Ylength+calculating_y_dis;\nelse\nYerror= Ylength-calculating_y_dis;\n\nif (calculating_y_dis>1000)\nstay=0;\nif (stay==0 )\nYerror=0;"("Ylength"=w55, "calculating_y_dis"=w67, "stay"=1) -> ("Yerror"=w127:dbl)
    n120 = Divide(x=w142, y=52.56) -> (x/y=→"p1 dis 2":dbl)
    n121 = formula code="X=((PulseM1/52.56)+(PulseM2/52.56))/2.0;\nY=((PulseM1/52.56)+(PulseM2/52.56))/2.0;"("PulseM1"=w138, "PulseM2"=w142) -> ("X"=w72:dbl, "Y"=w76:dbl)
    n122 = local read "check instruc"() -> (w58:bool)
    n123 = Multiply(x=1000, y=w76) -> (x*y=w79:dbl)
    n124 = xnode "PID"("Error"=w127) -> ("Output"=w78:dbl)  [unwired: 2 in, 11 out]
    n125 = local read "x check"() -> (w59:dbl)
    n126 = Select(t=w59, s=w58, f="X Length") -> (s? t:f=w56:dbl)
    n127 = Multiply(x=w56, y=10) -> (x*y=w63:dbl)
    "x entered" <- w63
    n128 = Multiply(x=1000, y=w72) -> (x*y=w73:dbl)
    n129 = Greater?(x=1, y=w78) -> (0:w91:bool)
    n130 = Less?(x=-1, y=w78) -> (x < y?=w89:bool)
    n131 = case shown="2000" w93 {
      tunnel: "motor 1" -> [w1031 w1034 w1037 w1044 w1048 w1052 w1058 w1064 w1070 w1075 w1082]
      tunnel: "motor 2" -> [w1028 w1036 w1039 w1042 w1047 w1050 w1056 w1062 w1068 w1076 w1081]
      tunnel: [w1027 w1036 w1038 w1041 w1047 w1049 w1055 w1061 w1067 w1073 w1080] -> w61
      tunnel: [w1030 w1033 w1037 w1043 w1048 w1051 w1057 w1063 w1069 w1074 w1079] -> w62
      frame 0, Default {
        n132 = Multiply(x=0, y=w1031) -> (x*y=w1030:dbl)
        n133 = Multiply(x=0, y=w1028) -> (x*y=w1027:dbl)
      }
      frame 1 {
        n134 = Multiply(x=-1, y=w1034) -> (x*y=w1033:dbl)
      }
      frame 2 {
        n135 = Multiply(x=-1.003, y=w1039) -> (x*y=w1038:dbl)
      }
      frame 10 {
        n136 = Multiply(x=-1, y=w1044) -> (x*y=w1043:dbl)
        n137 = Multiply(x=-1.1, y=w1042) -> (x*y=w1041:dbl)
      }
      frame 20 {
      }
      frame 100 {
        n138 = Multiply(x=0, y=w1052) -> (x*y=w1051:dbl)
        n139 = Multiply(x=1, y=w1050) -> (x*y=w1049:dbl)
      }
      frame 200 {
        n140 = Multiply(x=0, y=w1058) -> (x*y=w1057:dbl)
        n141 = Multiply(x=-1, y=w1056) -> (x*y=w1055:dbl)
      }
      frame 1000 {
        n142 = Multiply(x=-1, y=w1064) -> (x*y=w1063:dbl)
        n143 = Multiply(x=0, y=w1062) -> (x*y=w1061:dbl)
      }
      frame 2000 {
        n144 = Multiply(x=1, y=w1070) -> (x*y=w1069:dbl)
        n145 = Multiply(x=0, y=w1068) -> (x*y=w1067:dbl)
      }
      frame 4000 {
        n146 = Multiply(x=-1, y=w1075) -> (x*y=w1074:dbl)
        n147 = Multiply(x=0, y=w1076) -> (x*y=w1073:dbl)
      }
      frame 8000 {
        n148 = Multiply(x=-1, y=w1082) -> (x*y=w1079:dbl)
        n149 = Multiply(x=0, y=w1081) -> (x*y=w1080:dbl)
      }
    }
    n150 = And(x=w91, y=w89) -> (x .and. y?=w77:bool)
    "reached y" <- w77
    n151 = Select(t=w79, s=w77, f=w76) -> (s? t:f=w75:dbl)
    n152 = feedback-in #2(w75) -> ()
    n153 = Multiply(x=0, y=w78) -> (x*y=w87:dbl)
    n154 = Select(t=w87, s=w77, f=w78) -> (s? t:f=→"error y":dbl)
    n155 = local read "Numeric"() -> (w131:dbl)
    n156 = Or(x=w160, y=w159) -> (x .or. y?=w203:bool)
    n157 = local read "Draw circle"() -> (w135:bool)
    n158 = local read "Draw rectangle"() -> (w134:bool)
    n159 = And(x=w158, y=w151) -> (x .and. y?=w132:bool)
    n160 = Exclusive Or(1:w151, 2:w158) -> (0:w165:bool)
    n161 = Select(t=1, s=w158, f=0) -> (s? t:f=w150:i32)
    n162 = Select(t=2, s=w151, f=w150) -> (s? t:f=w155:i32)
    n163 = Select(t=1, s=w165, f=w131) -> (s? t:f=w164:dbl)
    n164 = Select(t=2, s=w132, f=w164) -> (s? t:f=w162:dbl)
    n165 = feedback #3() -> (w70:bool)  [unwired: 1 in]
    "reached x" <- w70
    n166 = Select(t=w73, s=w70, f=w72) -> (s? t:f=w66:dbl)
    "calc distanc x" <- w66
    n167 = formula code="if (desired_xlength==0)\nXerror=0;\nelse\nif(desired_xlength>0)\nXerror=desired_xlength-actual_xLength;\nelse\nXerror=desired_xlength+actual_xLength;\n\nif (actual_xLength>1000)\nstay1=0;\nif (stay1==0)\nXerror=0;"("actual_xLength"=w66, "desired_xlength"=w63, "stay1"=1) -> ("Xerror"=w126:dbl)
    "error calced" <- w126
    n168 = xnode "PID 2"("Error"=w126) -> ("Output"=w82:dbl)  [unwired: 2 in, 11 out]
    n169 = Greater?(x=1, y=w82) -> (0:w68:bool)
    "greater -1 x" <- w68
    n170 = Less?(x=-1, y=w82) -> (x < y?=w69:bool)
    "less 1 x" <- w69
    n171 = And(x=w68, y=w69) -> (x .and. y?=w71:bool)
    n172 = Multiply(x=0, y=w82) -> (x*y=w84:dbl)
    n173 = feedback-in #3(w71) -> ()
    n174 = Or(x=w135, y=w134) -> (x .or. y?=w136:bool)
    n175 = Select(t=w84, s=w70, f=w82) -> (s? t:f=→"error x":dbl)
    n176 = call "Number To Enum.vim"("number"=w155, "enum type"=enum16{"Nothing", "Left", "Top"}."Nothing") -> ("number as enum"=w152:enum16{"Nothing", "Left", "Top"})
    n177 = case shown="True" w149 {
      selector: w149 -> [w823 w831]
      tunnel: [w823 w831] -> w166
      tunnel: w152 -> [_ w824]
      frame False {
        n178 = local write "x distance currently being travelled"(0) -> ()
        n179 = local write "y distance currently being travelled"(0) -> ()
      }
      frame True {
        n180 = local read "Numeric"() -> (w829:dbl)
        n181 = local read "Shape drawing steps"() -> (w826:enum16{"corner", "1st switch", "reverse"})
        n182 = Equal?(x=w829, y=2) -> (x = y?=w828:bool)
        n183 = Select(t=enum16{"corner", "1st switch", "reverse"}."reverse", s=w828, f=w826) -> (s? t:f=w825:enum16{"corner", "1st switch", "reverse"})
        n184 = case shown="\"reverse\"" w825 {
          tunnel: w824 -> [_ w835 _]
          frame "corner" {
            n185 = local write "Has encoders been reset?"(enum16{"don't reset", "reset"}."don't reset") -> ()
            n186 = local write "y distance currently being travelled"(50) -> ()
            n187 = local write "x distance currently being travelled"(-50) -> ()
          }
          frame "1st switch" {
            n188 = local write "Has encoders been reset?"(enum16{"don't reset", "reset"}."don't reset") -> ()
            n189 = case shown="\"Top\"" w835 {
              frame "Nothing", Default {
                n190 = local write "y distance currently being travelled"(0) -> ()
                n191 = local write "x distance currently being travelled"(0) -> ()
                n192 = local write "Numeric"(2) -> ()
              }
              frame "Left" {
                n193 = local write "x distance currently being travelled"(0) -> ()
                n194 = local write "y distance currently being travelled"(50) -> ()
              }
              frame "Top" {
                n195 = local write "y distance currently being travelled"(0) -> ()
                n196 = local write "x distance currently being travelled"(-50) -> ()
              }
            }
          }
          frame "reverse" {
            n197 = local read "Draw circle"() -> (w844:bool)
            n198 = case shown="False" w844 {
              tunnel: "part" -> [w847 _]
              frame False {
                n199 = case shown="\"b\"" w847 {
                  frame "a" {
                    n200 = for {
                      N: 1 -> [_]
                      n201 = local read "Draw rectangle"() -> (w851:bool)
                      n202 = local write "Has encoders been reset?"(enum16{"don't reset", "reset"}."reset") -> ()
                      n203 = local read "Pulses M1"() -> (w860:dbl)
                      n204 = Select(t=TRUE, s=w851, f=FALSE) -> (s? t:f=w854:bool)
                      n205 = Equal To 0?(x=w860) -> (x = 0?=w853:bool)
                      n206 = And(x=w854, y=w853) -> (x .and. y?=w852:bool)
                      n207 = Select(t=T2."b", s=w852, f=T2."a") -> (s? t:f=w859:T2)
                      n208 = local write "part"(w859) -> ()
                      "Step 2A" <- TRUE
                    }
                    n209 = local write "y distance currently being travelled"(0) -> ()
                    n210 = local write "x distance currently being travelled"(0) -> ()
                  }
                  frame "b" {
                    n211 = local read "calc distance y"() -> (w863:dbl)
                    n212 = local read "calc distanc x"() -> (w864:dbl)
                    n213 = local write "Has encoders been reset?"(enum16{"don't reset", "reset"}."don't reset") -> ()
                    n214 = Greater?(x=w863, y=9000) -> (0:w869:bool)
                    n215 = Greater?(x=w864, y=29000) -> (0:w868:bool)
                    n216 = And(x=w868, y=w869) -> (x .and. y?=w867:bool)
                    "c" <- w867
                    n217 = Select(t=T2."c", s=w867, f=T2."b") -> (s? t:f=w872:T2)
                    n218 = local write "part"(w872) -> ()
                    "x distance currently being travelled" <- 3
                    "y distance currently being travelled" <- 1
                    "Step 2B" <- TRUE
                  }
                  frame "c" {
                    n219 = for {
                      N: 1 -> [_]
                      n220 = local read "Pulses M1"() -> (w888:dbl)
                      n221 = local read "Pulses M2"() -> (w884:dbl)
                      n222 = local write "Has encoders been reset?"(enum16{"don't reset", "reset"}."reset") -> ()
                      n223 = Equal To 0?(x=w884) -> (x = 0?=w882:bool)
                      n224 = Equal To 0?(x=w888) -> (x = 0?=w883:bool)
                      n225 = And(x=w883, y=w882) -> (x .and. y?=w881:bool)
                      n226 = Select(t=T2."d", s=w881, f=T2."c") -> (s? t:f=w887:T2)
                      n227 = local write "part"(w887) -> ()
                    }
                    n228 = local write "y distance currently being travelled"(0) -> ()
                    n229 = local write "x distance currently being travelled"(0) -> ()
                    "Step 2C" <- TRUE
                  }
                  frame "d" {
                    n230 = local write "Has encoders been reset?"(enum16{"don't reset", "reset"}."don't reset") -> ()
                    n231 = Multiply(x="height", y=10000) -> (x*y=w897:dbl)
                    n232 = local write "y distance currently being travelled"("height") -> ()
                    n233 = local write "x distance currently being travelled"(0) -> ()
                    n234 = Subtract(x=w897, y=1) -> (x-y=w894:dbl)
                    n235 = local read "calc distance y"() -> (w899:dbl)
                    n236 = Greater?(x=w899, y=w894) -> (0:w890:bool)
                    "Step 2D" <- w890
                    n237 = Select(t=T2."e", s=w890, f=T2."d") -> (s? t:f=w900:T2)
                    n238 = local write "part"(w900) -> ()
                  }
                  frame "e" {
                    n239 = local write "y distance currently being travelled"(0) -> ()
                    n240 = local write "x distance currently being travelled"(0) -> ()
                    n241 = for {
                      N: 1 -> [_]
                      n242 = local read "Pulses M2"() -> (w906:dbl)
                      n243 = local read "Pulses M1"() -> (w907:dbl)
                      n244 = local write "Has encoders been reset?"(enum16{"don't reset", "reset"}."reset") -> ()
                      n245 = Equal To 0?(x=w906) -> (x = 0?=w912:bool)
                      n246 = Equal To 0?(x=w907) -> (x = 0?=w913:bool)
                      n247 = And(x=w913, y=w912) -> (x .and. y?=w911:bool)
                      n248 = Select(t=T2."f", s=w911, f=T2."e") -> (s? t:f=w905:T2)
                      n249 = local write "part"(w905) -> ()
                    }
                  }
                  frame "f" {
                    n250 = Multiply(x="length", y=10000) -> (x*y=w920:dbl)
                    n251 = local read "calc distanc x"() -> (w923:dbl)
                    n252 = Subtract(x=w920, y=1) -> (x-y=w917:dbl)
                    n253 = local write "Has encoders been reset?"(enum16{"don't reset", "reset"}."don't reset") -> ()
                    n254 = local write "x distance currently being travelled"("length") -> ()
                    n255 = Greater?(x=w923, y=w917) -> (0:w914:bool)
                    "at 2f" <- w914
                    n256 = local write "y distance currently being travelled"(0) -> ()
                    n257 = Select(t=T2."g", s=w914, f=T2."f") -> (s? t:f=w922:T2)
                    n258 = local write "part"(w922) -> ()
                  }
                  frame "g" {
                    n259 = local write "y distance currently being travelled"(0) -> ()
                    n260 = local write "x distance currently being travelled"(0) -> ()
                    n261 = for {
                      N: 1 -> [_]
                      n262 = local read "Pulses M1"() -> (w930:dbl)
                      n263 = local read "Pulses M2"() -> (w929:dbl)
                      n264 = local write "Has encoders been reset?"(enum16{"don't reset", "reset"}."reset") -> ()
                      n265 = Equal To 0?(x=w929) -> (x = 0?=w936:bool)
                      n266 = Equal To 0?(x=w930) -> (x = 0?=w937:bool)
                      n267 = And(x=w937, y=w936) -> (x .and. y?=w935:bool)
                      n268 = Select(t=T2."h", s=w935, f=T2."g") -> (s? t:f=w932:T2)
                      n269 = local write "part"(w932) -> ()
                    }
                  }
                  frame "h" {
                    n270 = local write "Has encoders been reset?"(enum16{"don't reset", "reset"}."don't reset") -> ()
                    n271 = local read "height"() -> (w941:dbl)
                    n272 = Multiply(x=w941, y=10000) -> (x*y=w949:dbl)
                    n273 = local write "y distance currently being travelled"(w941) -> ()
                    n274 = Subtract(x=w949, y=1) -> (x-y=w946:dbl)
                    n275 = local write "x distance currently being travelled"(0) -> ()
                    n276 = local read "calc distance y"() -> (w939:dbl)
                    n277 = Greater?(x=w939, y=w946) -> (0:w950:bool)
                    n278 = Select(t=T2."i", s=w950, f=T2."h") -> (s? t:f=w942:T2)
                    n279 = local write "part"(w942) -> ()
                    "Step 2H" <- TRUE
                  }
                  frame "i" {
                    n280 = for {
                      N: 1 -> [_]
                      n281 = local read "Pulses M1"() -> (w956:dbl)
                      n282 = local read "Pulses M2"() -> (w955:dbl)
                      n283 = local write "Has encoders been reset?"(enum16{"don't reset", "reset"}."reset") -> ()
                      n284 = Equal To 0?(x=w955) -> (x = 0?=w961:bool)
                      n285 = Equal To 0?(x=w956) -> (x = 0?=w962:bool)
                      n286 = And(x=w962, y=w961) -> (x .and. y?=w960:bool)
                      n287 = Select(t=T2."j", s=w960, f=T2."i") -> (s? t:f=w954:T2)
                      n288 = local write "part"(w954) -> ()
                    }
                    n289 = local write "y distance currently being travelled"(0) -> ()
                    n290 = local write "x distance currently being travelled"(0) -> ()
                  }
                  frame "j" {
                    (unwired) 1
                    n291 = local read "length"() -> (w966:dbl)
                    n292 = local read "calc distanc x"() -> (w968:dbl)
                    n293 = Multiply(x=w966, y=10000) -> (x*y=w963:dbl)
                    n294 = local write "Has encoders been reset?"(enum16{"don't reset", "reset"}."don't reset") -> ()
                    n295 = local write "x distance currently being travelled"(w966) -> ()
                    n296 = Greater?(x=w968, y=w963) -> (0:w971:bool)
                    n297 = local write "y distance currently being travelled"(0) -> ()
                    n298 = Select(t=T2."nothing", s=w971, f=T2."j") -> (s? t:f=w967:T2)
                    n299 = local write "part"(w967) -> ()
                    "Step 2J" <- TRUE
                  }
                  frame "nothing" {
                    n300 = local write "y distance currently being travelled"(0) -> ()
                    n301 = local write "x distance currently being travelled"(0) -> ()
                  }
                }
              }
              frame True {
                n302 = case shown="\"radius_travel\"" "part circle" {
                  frame "a" {
                    n303 = for {
                      N: 1 -> [_]
                      n304 = local read "Pulses M1"() -> (w985:dbl)
                      n305 = local read "Pulses M2"() -> (w984:dbl)
                      n306 = Equal To 0?(x=w985) -> (x = 0?=w987:bool)
                      n307 = Equal To 0?(x=w984) -> (x = 0?=w988:bool)
                      n308 = And(x=w987, y=w988) -> (x .and. y?=w986:bool)
                      "circle reset" <- w986
                      n309 = Select(t=T1."going right", s=w986, f=T1."a") -> (s? t:f=w982:T1)
                      n310 = local write "Has encoders been reset?"(enum16{"don't reset", "reset"}."reset") -> ()
                      n311 = local write "part circle"(w982) -> ()
                    }
                    n312 = local write "x distance currently being travelled"(0) -> ()
                    n313 = local write "y distance currently being travelled"(0) -> ()
                  }
                  frame "going down" {
                    n314 = local read "calc distance y"() -> (w997:dbl)
                    n315 = Greater?(x=w997, y=19000) -> (0:w995:bool)
                    n316 = local write "Has encoders been reset?"(enum16{"don't reset", "reset"}."don't reset") -> ()
                    n317 = Select(t=T1."going right", s=w995, f=T1."going down") -> (s? t:f=w992:T1)
                    n318 = local write "y distance currently being travelled"(-2) -> ()
                    n319 = local write "x distance currently being travelled"(0) -> ()
                    n320 = local write "part circle"(w992) -> ()
                    "down" <- TRUE
                  }
                  frame "going right" {
                    n321 = for {
                      N: 1 -> [_]
                      n322 = local read "Pulses M1"() -> (w1008:dbl)
                      n323 = local read "Pulses M2"() -> (w1007:dbl)
                      n324 = Equal To 0?(x=w1008) -> (x = 0?=w1010:bool)
                      n325 = Equal To 0?(x=w1007) -> (x = 0?=w1011:bool)
                      n326 = And(x=w1010, y=w1011) -> (x .and. y?=w1009:bool)
                      n327 = Select(t=T1."radius_travel", s=w1009, f=T1."going right") -> (s? t:f=w1005:T1)
                      n328 = local write "Has encoders been reset?"(enum16{"don't reset", "reset"}."reset") -> ()
                      n329 = local write "part circle"(w1005) -> ()
                    }
                    n330 = local write "x distance currently being travelled"(0) -> ()
                    n331 = local write "y distance currently being travelled"(0) -> ()
                    "right" <- TRUE
                  }
                  frame "radius_travel" {
                    n332 = local read "calc distanc x"() -> (w1014:dbl)
                    n333 = local write "x distance currently being travelled"(-4) -> ()
                    n334 = Greater?(x=w1014, y=39000) -> (0:w1018:bool)
                    n335 = local write "Has encoders been reset?"(enum16{"don't reset", "reset"}."don't reset") -> ()
                    n336 = Select(t=T1."going right", s=w1018, f=T1."going down") -> (s? t:f=w1013:T1)
                    n337 = local write "part circle"(w1013) -> ()
                    "down 2" <- TRUE
                  }
                  frame "reset_before_circle" {
                    n338 = local write "x distance currently being travelled"(0) -> ()
                    n339 = local write "y distance currently being travelled"(0) -> ()
                  }
                  frame "circle" {
                    n340 = local write "x distance currently being travelled"(0) -> ()
                    n341 = local write "y distance currently being travelled"(0) -> ()
                  }
                  frame "nothing" {
                    n342 = local write "x distance currently being travelled"(0) -> ()
                    n343 = local write "y distance currently being travelled"(0) -> ()
                  }
                }
              }
            }
            "Numeric" <- 2
          }
        }
      }
    }
    "In drawing mode" <- w166
    n344 = And(x=w77, y=w70) -> (x .and. y?=w148:bool)
    n345 = Or(x=w203, y=w148) -> (x .or. y?=w202:bool)
    n346 = Or(x=w202, y="Motor stop") -> (x .or. y?=w204:bool)
    n347 = Or(x=w204, y="stop") -> (x .or. y?=w224:bool)
    n348 = Select(t=0.0, s=w224, f=w61) -> (s? t:f=w221:dbl)
    n349 = call-poly <vilib>:"DAQmx Write.vi"("task/channels in"=w230, "data"=w221, "error in"=w227) -> ("task out"=w231:refnum<k21>, "error out"=w232:errorcluster)  [unwired: 10 in, 1 out]
    n350 = Select(t=0.0 ("s? t:f"), s=w224, f=w62) -> (s? t:f=w222:dbl)
    n351 = call-poly <vilib>:"DAQmx Write.vi"("task/channels in"=w236, "data"=w222, "error in"=w226) -> ("task out"=w235:refnum<k21>, "error out"=w234:errorcluster)  [unwired: 10 in, 1 out]
    n352 = call <vilib>:"DAQmx Wait Until Done.vi"("task/channels in"=w235, "error in"=w234) -> ("error out"=w233:errorcluster)  [unwired: 12 in, 1 out]
    n353 = call <vilib>:"DAQmx Wait Until Done.vi"("task/channels in"=w231, "error in"=w232) -> ("error out"=w229:errorcluster)  [unwired: 12 in, 1 out]
    n354 = case shown="True" w136 {
      tunnel: w137 -> [w298 w299]
      frame False {
        n355 = call-poly <vilib>:"DAQmx Read.vi"("task/channels in"=w298) -> ("data"=w297:dbl)  [unwired: 12 in, 2 out]
        n356 = local write "Pulses M2"(w297) -> ()
      }
      frame True {
        n357 = local read "Has encoders been reset?"() -> (w300:enum16{"don't reset", "reset"})
        n358 = case shown="\"reset\"" w300 {
          tunnel: w299 -> [w302 w305]
          frame "don't reset", Default {
            n359 = call-poly <vilib>:"DAQmx Read.vi"("task/channels in"=w302) -> ("data"=→"Pulses M2":dbl)  [unwired: 12 in, 2 out]
          }
          frame "reset" {
            n360 = call <vilib>:"DAQmx Stop Task.vi"("task/channels in"=w305) -> ("task out"=w304:refnum<k21>)  [unwired: 13 in, 1 out]
            n361 = call <vilib>:"DAQmx Start Task.vi"("task/channels in"=w304) -> ("task out"=w306:refnum<k21>)  [unwired: 13 in, 1 out]
            n362 = call-poly <vilib>:"DAQmx Read.vi"("task/channels in"=w306) -> ("data"=w303:dbl)  [unwired: 12 in, 2 out]
            n363 = local write "Pulses M2"(w303) -> ()
          }
        }
      }
    }
    n364 = call "Number To Enum.vim"("number"=w162, "enum type"=enum16{"corner", "1st switch", "reverse"}."corner") -> ("number as enum"=→"Shape drawing steps":enum16{"corner", "1st switch", "reverse"})
    n365 = case shown="True" w136 {
      tunnel: w141 -> [w309 w314]
      tunnel: w140 -> [w310 w313]
      tunnel: [w307 w312] -> w139
      frame False {
        n366 = call-poly <vilib>:"DAQmx Read.vi"("task/channels in"=w309, "error in"=w310) -> ("data"=w308:dbl, "error out"=w307:errorcluster)  [unwired: 11 in, 1 out]
        n367 = local write "Pulses M1"(w308) -> ()
      }
      frame True {
        n368 = case shown="\"reset\"" "Has encoders been reset?" {
          tunnel: w314 -> [w318 w325]
          tunnel: w313 -> [w317 w324]
          tunnel: [w315 w326] -> w312
          frame "don't reset", Default {
            n369 = call-poly <vilib>:"DAQmx Read.vi"("task/channels in"=w318, "error in"=w317) -> ("data"=→"Pulses M1":dbl, "error out"=w315:errorcluster)  [unwired: 11 in, 1 out]
          }
          frame "reset" {
            n370 = call <vilib>:"DAQmx Stop Task.vi"("task/channels in"=w325, "error in"=w324) -> ("task out"=w323:refnum<k21>, "error out"=w322:errorcluster)  [unwired: 12 in]
            n371 = call <vilib>:"DAQmx Start Task.vi"("task/channels in"=w323, "error in"=w322) -> ("task out"=w321:refnum<k21>, "error out"=w320:errorcluster)  [unwired: 12 in]
            n372 = call-poly <vilib>:"DAQmx Read.vi"("task/channels in"=w321, "error in"=w320) -> ("data"=w319:dbl, "error out"=w326:errorcluster)  [unwired: 11 in, 1 out]
            n373 = local write "Pulses M1"(w319) -> ()
          }
        }
      }
    }
  }
  n374 = invoke on="motor 1" class="Slide (strict)" method="Reinit To Default"() -> ()  [unwired: 3 in, 3 out]
  n375 = call <vilib>:"Simple Error Handler.vi"("error source (\" \")"="you messed up" ("error source (\" \")"), "error in (no error)"=w48) -> ()  [unwired: 3 in, 5 out]
  n376 = call <vilib>:"Simple Error Handler.vi"("error source (\" \")"="you messed up" ("error source (\" \")"), "error in (no error)"=w45) -> ()  [unwired: 3 in, 5 out]
  n377 = call <vilib>:"DAQmx Clear Task.vi"("task in"=w27, "error in"=w25) -> ()  [unwired: 13 in, 1 out]
  n378 = call <vilib>:"DAQmx Clear Task.vi"("task in"=w17, "error in"=w14) -> ()  [unwired: 13 in, 1 out]
  n379 = call <vilib>:"DAQmx Clear Task.vi"("task in"=w18, "error in"=w15) -> ("error out"=w12:errorcluster)  [unwired: 13 in]
  n380 = call <vilib>:"DAQmx Clear Task.vi"("task in"=w16, "error in"=w13) -> ()  [unwired: 13 in, 1 out]
  n381 = call <vilib>:"Simple Error Handler.vi"("error in (no error)"=w12) -> ()  [unwired: 4 in, 5 out]
  n382 = call <vilib>:"Simple Error Handler.vi"("error source (\" \")"="you messed up" ("error source (\" \")"), "error in (no error)"=w10) -> ()  [unwired: 3 in, 5 out]
